vi "Untitled 1.vi"() -> ()   [LabVIEW 2017]
panel:
  out "resulting string":string
  in  "brake control":bool
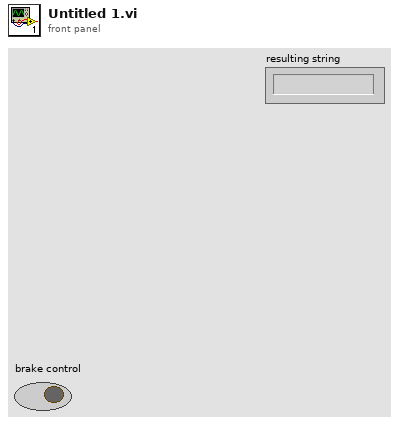
[diagram p1: front panel]
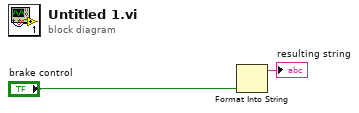
[diagram p0: block diagram]
diagram:
  n1 = Format Into String("brake control") -> (resulting string=→"resulting string":string)  [unwired: 3 in, 1 out]
